vi "testlimits.vi"() -> ()   [LabVIEW 2014]
panel:
  out "error out":errorcluster
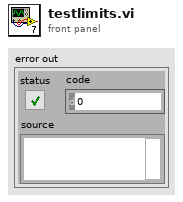
[diagram p1: front panel]
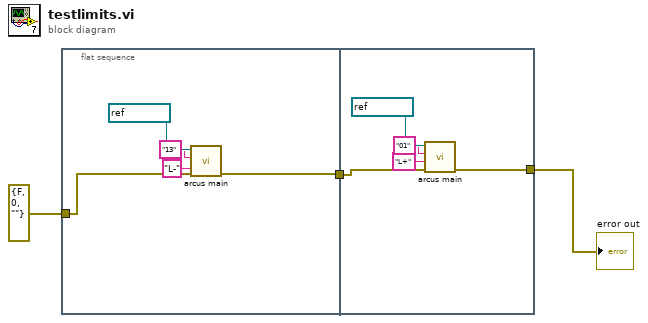
[diagram p0: block diagram]
diagram:
  n1 = flat-sequence {
    tunnel: errorcluster {"status"=FALSE, "code"=0, "source"=""} ("error in (no error)") -> [w8]
    tunnel: [w7] -> w2
    tunnel: w2 -> [w13]
    tunnel: [w12] -> w1
    frame #0 {
      n2 = call "arcus main.vi"("Communication Port"=refnum<visa-resource-name> "COM4", "Device Address"="13", "Command"="L-", "error in (no error)"=w8) -> ("error out"=w7:errorcluster)  [unwired: 5 in, 1 out]
    }
    frame #1 {
      n3 = call "arcus main.vi"("Communication Port"=refnum<visa-resource-name> "COM4", "Device Address"="01", "Command"="L+", "error in (no error)"=w13) -> ("error out"=w12:errorcluster)  [unwired: 5 in, 1 out]
    }
  }
  "error out" <- w1
